vi "RaiseElevator.vi"(11 "Distance":dbl) -> ()   [LabVIEW 2015]
uses:
  Robot Global Data.vi
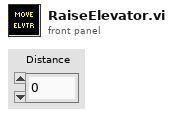
[diagram p1: front panel]
types:
  T1 = typedef "WPI_PotentiometerDevRef.ctl" = cluster{"DevStatus":errorcluster, "Analog Channel":T2, "Invert Output":bool}
  T2 = typedef "FPGA_AIChannel.ctl" = enum8{"AI 0", "AI 1", "AI 2", "AI 3", "AI MXP 0", "AI MXP 1", "AI MXP 2", "AI MXP 3", "Invalid"}
  T3 = typedef "WPI_MotorControlDeviceRef.ctl" = cluster{"DeviceStatus":errorcluster, "Type":T4, "PWM":cluster{"PWM Channel":T5, "DeadBand":T6}, "CAN":cluster{"Device Number":u8, "Control Mode":T7, "Semaphore":T8, "Max Vout":dbl, "TalonSRX Control Mode":T9}, "Invert":bool}
  T4 = typedef "WPI_MotorControlType.ctl" = enum16{"PWM", "CAN", "CANTalonSRX"}
  T5 = typedef "FPGA_DIOPWMChannel.ctl" = enum8{"PWM 0", "PWM 1", "PWM 2", "PWM 3", "PWM 4", "PWM 5", "PWM 6", "PWM 7", "PWM 8", "PWM 9", "PWM MXP 0", "PWM MXP 1", "PWM MXP 2", "PWM MXP 3", "PWM MXP 4", "PWM MXP 5", "PWM MXP 6", "PWM MXP 7", "PWM MXP 8", "PWM MXP 9", "Invalid"}
  T6 = typedef "WPI_PWMDeadband.ctl" = cluster{"Name":string, "maxPositivePwm":i32, "minPositivePwm":i32, "centerPwm":i32, "maxNegativePwm":i32, "minNegativePwm":i32, "angularRange":u16}
  T7 = typedef "WPI_CANJaguar_ControlMode.ctl" = enum8{"Percent VBus", "Current", "Speed", "Position", "Voltage"}
  T8 = typedef "Semaphore RefNum" = refnum<k1>
  T9 = typedef "WPI_CANTalonSRX_APIControlMode.ctl" = enum8{"Percent VBus", "Speed", "Position", "Slave", "Unchanged / Invalid", "Voltage Compensation", "Current", "Motion Profile"}
  T10 = typedef "WPI_SwitchDevRef.ctl" = cluster{"DevStatus":errorcluster, "DIO Channel":T11, "CntIndex":T12, "Normally Closed":bool}
  T11 = typedef "FPGA_DIOChannel.ctl" = enum8{"DIO 0", "DIO 1", "DIO 2", "DIO 3", "DIO 4", "DIO 5", "DIO 6", "DIO 7", "DIO 8", "DIO 9", "DIO MXP 0", "DIO MXP 1", "DIO MXP 2", "DIO MXP 3", "DIO MXP 4", "DIO MXP 5", "DIO MXP 6", "DIO MXP 7", "DIO MXP 8", "DIO MXP 9", "DIO MXP 10", "DIO MXP 11", "DIO MXP 12", "DIO MXP 13", "DIO MXP 14", "DIO MXP 15", "Invalid"}
  T12 = typedef "FPGA_CounterCtrSystemIndex.ctl" = enum8{"Ctr 0", "Ctr 1", "Ctr 2", "Ctr 3", "Ctr 4", "Ctr 5", "Ctr 6", "Ctr 7", "Invalid"}
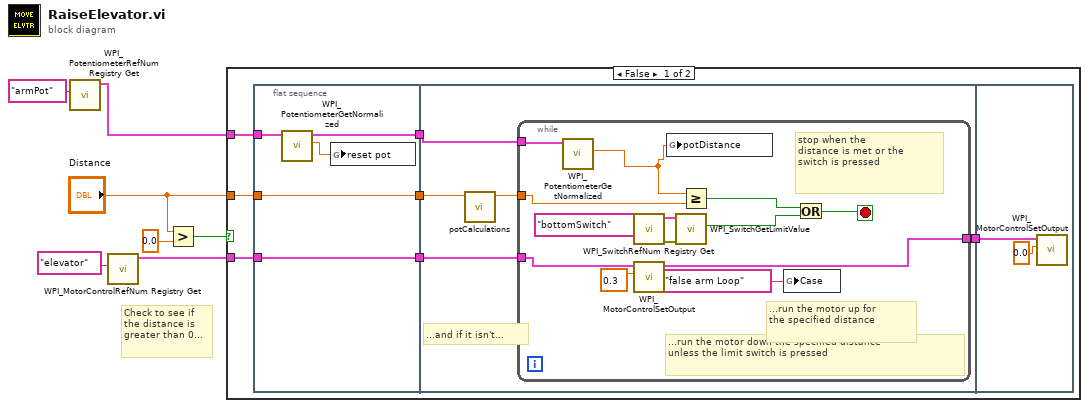
[diagram p0: block diagram]
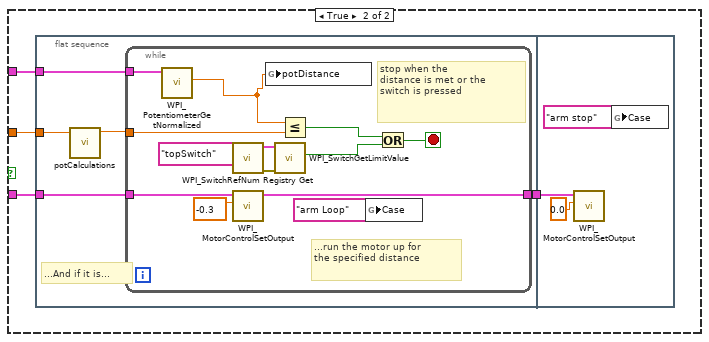
[diagram p2: hidden frame]
diagram:
  # "Check to see if\nthe distance is\ngreater than 0..."
  n1 = call <vilib>:"WPI_PotentiometerRefNum Registry Get.vi"("refnum name"="armPot") -> ("PotDevRef"=w2:T1)  [unwired: 9 in, 1 out]
  n2 = call <vilib>:"WPI_MotorControlRefNum Registry Get.vi"("refnum name"="elevator") -> ("MotorControlDevRef"=w6:T3)  [unwired: 9 in, 1 out]
  n3 = Greater?(x="Distance", y=0.0) -> (0:w5:bool)
  n4 = case shown="False" w5 {
    tunnel: "Distance" -> [w13 w42]
    tunnel: w6 -> [w14 w43]
    tunnel: w2 -> [w12 w41]
    frame False {
      n5 = flat-sequence {
        tunnel: w12 -> [w17]
        tunnel: w13 -> [w18]
        tunnel: w14 -> [w19]
        tunnel: [w19] -> w10
        tunnel: [w18] -> w9
        tunnel: [w16] -> w8
        tunnel: [w20] -> w11
        tunnel: w10 -> [w24]
        tunnel: w9 -> [w22]
        tunnel: w8 -> [w23]
        tunnel: w11 -> [w38]
        frame #0 {
          n6 = call <vilib>:"WPI_PotentiometerGetNormalized.vi"("PotDevRef"=w17) -> ("Normalized Value"=w15:dbl, "PotDevRef"=w16:T1)  [unwired: 8 in, 1 out]
          n7 = global write "Robot Global Data.vi" "reset pot"(w15) -> ()
        }
        frame #1 {
          # "...and if it isn't..."
          n8 = call "potCalculations.vi"("Voltage in"=w22) -> ("distance out"=w21:dbl)  [unwired: 10 in]
          n9 = while {
            tunnel: w21 -> [w26]
            tunnel: w24 -> [w27]
            tunnel: w23 -> [w25]
            tunnel: [w28] -> w20
            stop <- w29 stop-if-true
            # "stop when the \ndistance is met or the\nswitch is pressed"
            # "...run the motor up for\nthe specified distance"
            # "...run the motor down the specified distance \nunless the limit switch is pressed"
            n10 = call <vilib>:"WPI_PotentiometerGetNormalized.vi"("PotDevRef"=w25) -> ("Normalized Value"=w30:dbl)  [unwired: 8 in, 2 out]
            n11 = call <vilib>:"WPI_SwitchRefNum Registry Get.vi"("refnum name"="bottomSwitch") -> ("error out"=w36:errorcluster, "SwitchDevRef"=w35:T10)  [unwired: 9 in]
            n12 = call <vilib>:"WPI_MotorControlSetOutput.vi"("Output"=0.3, "MotorControlDevRef"=w27) -> ("MotorControlDevRef"=w28:T3)  [unwired: 7 in, 2 out]
            n13 = global write "Robot Global Data.vi" "potDistance"(w30) -> ()
            n14 = call <vilib>:"WPI_SwitchGetLimitValue.vi"("error in (no error)"=w36, "SwitchDevRef"=w35) -> ("Switch Pressed"=w33:bool)  [unwired: 7 in, 2 out]
            n15 = Greater Or Equal?(x=w30, y=w26) -> (x >= y?=w32:bool)
            n16 = global write "Robot Global Data.vi" "Case"("false arm Loop" ("Case")) -> ()
            n17 = Or(x=w32, y=w33) -> (x .or. y?=w29:bool)
          }
        }
        frame #2 {
          n18 = call <vilib>:"WPI_MotorControlSetOutput.vi"("Output"=0.0, "MotorControlDevRef"=w38) -> ()  [unwired: 7 in, 3 out]
        }
      }
    }
    frame True {
      n19 = flat-sequence {
        tunnel: w43 -> [w48]
        tunnel: w42 -> [w45]
        tunnel: w41 -> [w47]
        tunnel: [w46] -> w40
        tunnel: w40 -> [w63]
        frame #0 {
          # "...And if it is..."
          n20 = call "potCalculations.vi"("Voltage in"=w45) -> ("distance out"=w44:dbl)  [unwired: 10 in]
          n21 = while {
            tunnel: w44 -> [w53]
            tunnel: w48 -> [w60]
            tunnel: w47 -> [w52]
            tunnel: [w50] -> w46
            stop <- w54 stop-if-true
            # "stop when the \ndistance is met or the\nswitch is pressed"
            # "...run the motor up for\nthe specified distance"
            n22 = call <vilib>:"WPI_PotentiometerGetNormalized.vi"("PotDevRef"=w52) -> ("Normalized Value"=w49:dbl)  [unwired: 8 in, 2 out]
            n23 = call <vilib>:"WPI_SwitchRefNum Registry Get.vi"("refnum name"="topSwitch") -> ("error out"=w59:errorcluster, "SwitchDevRef"=w58:T10)  [unwired: 9 in]
            n24 = call <vilib>:"WPI_MotorControlSetOutput.vi"("Output"=-0.3, "MotorControlDevRef"=w60) -> ("MotorControlDevRef"=w50:T3)  [unwired: 7 in, 2 out]
            n25 = global write "Robot Global Data.vi" "potDistance"(w49) -> ()
            n26 = call <vilib>:"WPI_SwitchGetLimitValue.vi"("error in (no error)"=w59, "SwitchDevRef"=w58) -> ("Switch Pressed"=w56:bool)  [unwired: 7 in, 2 out]
            n27 = Less Or Equal?(x=w49, y=w53) -> (x <= y?=w55:bool)
            n28 = global write "Robot Global Data.vi" "Case"("arm Loop" ("Case")) -> ()
            n29 = Or(x=w55, y=w56) -> (x .or. y?=w54:bool)
          }
        }
        frame #1 {
          n30 = call <vilib>:"WPI_MotorControlSetOutput.vi"("Output"=0.0, "MotorControlDevRef"=w63) -> ()  [unwired: 7 in, 3 out]
          n31 = global write "Robot Global Data.vi" "Case"("arm stop" ("Case")) -> ()
        }
      }
    }
  }
